vi "Decrement.vi"(8 "error in (no error)":errorcluster, 10 "Decrement by":dbl=1.0, 11 "Counter in":refnum<class "Counter.lvclass">) -> (0 "error out":errorcluster, 3 "Counter out":refnum<class "Counter.lvclass">)   [LabVIEW 2018, in "Counter.lvlib" / "Counter.lvclass"]
uses:
  Counter.lvclass
  Counter.lvclass/Counter.ctl
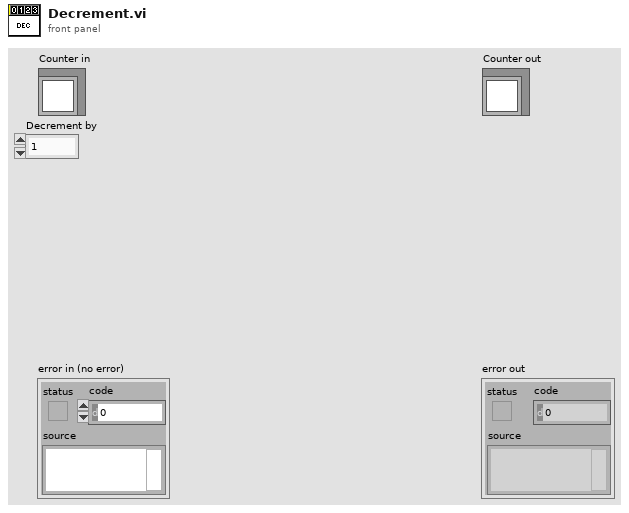
[diagram p1: front panel]
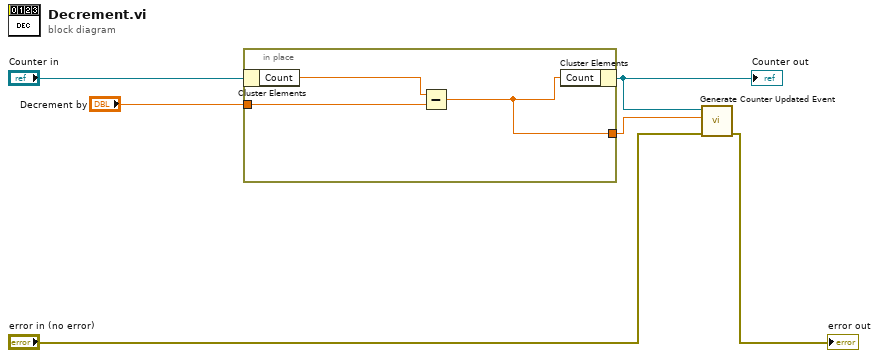
[diagram p0: block diagram]
diagram:
  n1 = in-place {
    in-place-border: "Decrement by" -> [w8]
    in-place-border: [w7] -> w3
    n2 = in-place-cluster #1("Counter in") -> ("Count"=w9:dbl)
    n3 = Subtract(x=w9, y=w8) -> (x-y=w7:dbl)
    n4 = in-place-cluster #1("Count"=w7) -> (w4:refnum<class "Counter.lvclass">)
  }
  "Counter out" <- w4
  n5 = call "Generate Counter Updated Event.vi"("error in (no error)"="error in (no error)", "Count"=w3, "Counter in"=w4) -> ("error out"=→"error out":errorcluster)  [unwired: 8 in]
